vi "Path-Find_Closest_Tile.vi"(9 "Goal":T1, 10 "Tiles":T1[](array[typedef])) -> (2 "Closest Tile":T1)   [LabVIEW 2020]
doc: "<B>Description:</B> Finds the tile closest to the goal.\n\n<B>Date:</B> 05/2019\n<B>Author:</B> Luke Jarocki, Choose Movement Consulting, LLC"
uses:
  Controls/Parse-(X,Y).ctl
  Controls/TileColor.ctl
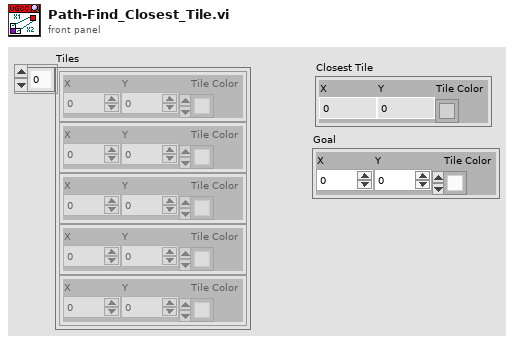
[diagram p1: front panel]
types:
  T1 = typedef "Parse-(X,Y).ctl" = cluster{"X":i32, "Y":i32, "Tile Color":T2}
  T2 = typedef "TileColor.ctl" = u16
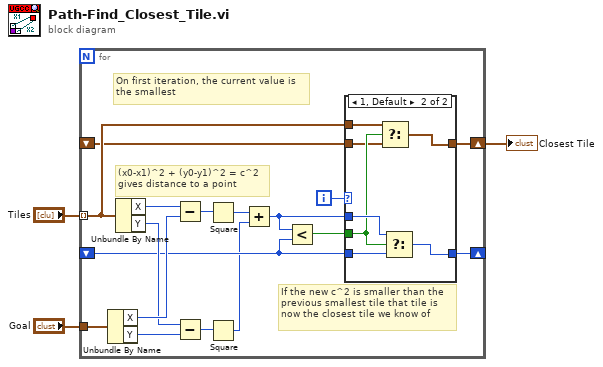
[diagram p0: block diagram]
diagram:
  n1 = for {
    tunnel: "Tiles" -> [w13] mode=indexing
    tunnel: "Goal" -> [w20]
    shift-right: [w15] -> _
    shift-left: _ -> [w8]
    shift-right: [w11] -> w1
    shift-left: _ -> [w12]
    i -> [w10]
    # "If the new c^2 is smaller than the\nprevious smallest tile that tile is\nnow the closest tile we know of"
    # "On first iteration, the current value is\nthe smallest"
    # "(x0-x1)^2 + (y0-y1)^2 = c^2\ngives distance to a point"
    n2 = Unbundle By Name(w20) -> ("X"=w18:i32, "Y"=w16:i32)
    n3 = Unbundle By Name(w13) -> ("X"=w19:i32, "Y"=w17:i32)
    n4 = Subtract(x=w19, y=w18) -> (x-y=w7:i32)
    n5 = Subtract(x=w17, y=w16) -> (x-y=w5:i32)
    n6 = Square(x=w7) -> (x^2=w4:i32)
    n7 = Square(x=w5) -> (x^2=w6:i32)
    n8 = Add(x=w4, y=w6) -> (x+y=w9:i32)
    n9 = Less?(x=w9, y=w8) -> (x < y?=w14:bool)
    n10 = case shown="1, Default" w10 {
      tunnel: w9 -> [w21 w29]
      tunnel: w8 -> [_ w28]
      tunnel: [w21 w27] -> w15
      tunnel: w14 -> [_ w26]
      tunnel: w13 -> [w22 w25]
      tunnel: w12 -> [_ w24]
      tunnel: [w22 w23] -> w11
      frame 0 {
      }
      frame 1, Default {
        n11 = Select(t=w25, s=w26, f=w24) -> (s? t:f=w23:T1)
        n12 = Select(t=w29, s=w26, f=w28) -> (s? t:f=w27:i32)
      }
    }
  }
  "Closest Tile" <- w1
